vi "update swerve odom.vi"(11 "Module Pos":T1[](array[typedef]) {"Angle"."SIN" format="%13.4f"; "Angle"."COS" format="%13.4f"; "Angle"."VALUE" format="%13.4f"}) -> ()   [LabVIEW 2020]
uses:
  <vilib>/Rock Robotics/WPI/ThirdParty/JAS_Junk/TrajLib/TypeDef/SWERVE_DRIVE_MODULE_POSITION.ctl
  <vilib>/Rock Robotics/WPI/ThirdParty/JAS_Junk/TrajLib/TypeDef/ROTATION2D.ctl
  Robot Global Data.vi
  <vilib>/Rock Robotics/WPI/ThirdParty/JAS_Junk/TrajLib/Trajectory_Library.lvlib
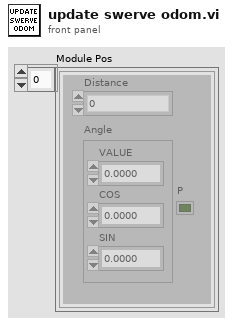
[diagram p1: front panel]
types:
  T1 = typedef "Trajectory_Library.lvlib/SWERVE_DRIVE_MODULE_POSITION.ctl" = cluster{"Distance":dbl, "Angle":T2, "P":bool}
  T2 = typedef "Trajectory_Library.lvlib/ROTATION2D.ctl" = cluster{"VALUE":dbl, "COS":dbl, "SIN":dbl}
  T3 = typedef "Trajectory_Library.lvlib/SWERVE_DRIVE_KINEMATICS.ctl" = cluster{"NumModules":i32, "InverseKinematics":T4, "ForwardKinematics":T4, "Modules":T5[], "PrevCoR":T5, "SavedModuleStates":T6[]}
  T4 = typedef "NI_Matrix.lvlib/RealMatrix.ctl" = dbl[][]
  T5 = typedef "Trajectory_Library.lvlib/TRANSLATION2D.ctl" = cluster{"X":dbl, "Y":dbl}
  T6 = typedef "Trajectory_Library.lvlib/SWERVE_DRIVE_MODULE_STATE.ctl" = cluster{"Speed":dbl, "Angle":T2}
  T7 = typedef "Trajectory_Library.lvlib/SWERVE_DRIVE_ODOMETRY.ctl" = cluster{"POSE":T8, "GyroOffset":T2, "PreviousAngle":T2, "PrevModulePositions":T1[], "NumModules":i32}
  T8 = typedef "Trajectory_Library.lvlib/POSE2D.ctl" = cluster{"TRANSLATION":T5, "ROTATION":T2}
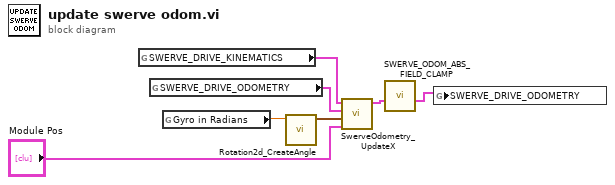
[diagram p0: block diagram]
diagram:
  n1 = global read "Robot Global Data.vi" "SWERVE_DRIVE_KINEMATICS"() -> (w4:T3)
  n2 = global read "Robot Global Data.vi" "SWERVE_DRIVE_ODOMETRY"() -> (w6:T7)
  n3 = global read "Robot Global Data.vi" "Gyro in Radians"() -> (w7:dbl)
  n4 = call <vilib>:"Rotation2d_CreateAngle.vi"("Angle"=w7) -> ("ROTATION"=w3:T2)  [unwired: 10 in]
  n5 = call <vilib>:"SwerveOdometry_UpdateX.vi"("module Positions"="Module Pos", "gyroAngle"=w3, "in SWERVE_DRIVE_ODOMETRY"=w6, "SWERVE_DRIVE_KINEMATICS"=w4) -> ("out SWERVE_DRIVE_ODOMETRY"=w2:T7)  [unwired: 5 in, 2 out]
  n6 = call "SWERVE_ODOM_ABS_FIELD_CLAMP.vi"("in SWERVE_DRIVE_ODOMETRY"=w2) -> ("out SWERVE_DRIVE_ODOMETRY"=w1:T7)  [unwired: 10 in]
  n7 = global write "Robot Global Data.vi" "SWERVE_DRIVE_ODOMETRY"(w1) -> ()
